vi "ReRouteAroundPolygon.vi"(2 "Desired Point Spacing (in)":dbl, 3 "AvoidancePolygon":T2, 4 "InputPath":T1[](array[typedef])) -> (0 "OutputPath":T1[](array[typedef]), 1 "PathChanged":bool)   [LabVIEW 2017, in "ArgosLib.lvlib"]
uses:
  ArgosLib.lvlib
  TypeDefs/Point2D.ctl
  TypeDefs/Polygon2D.ctl
panel:
  out "Paths":cluster{dbl[], dbl[]}[](graph)
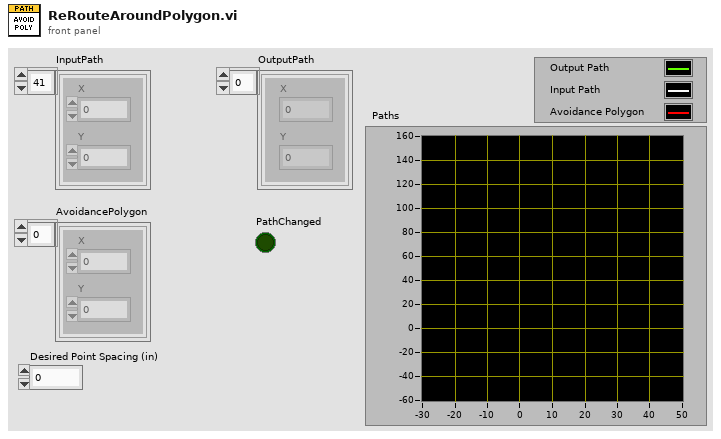
[diagram p1: front panel]
types:
  T1 = typedef "ArgosLib.lvlib/Point2D.ctl" = cluster{"X":dbl, "Y":dbl}
  T2 = typedef "ArgosLib.lvlib/Polygon2D.ctl" = T1[]
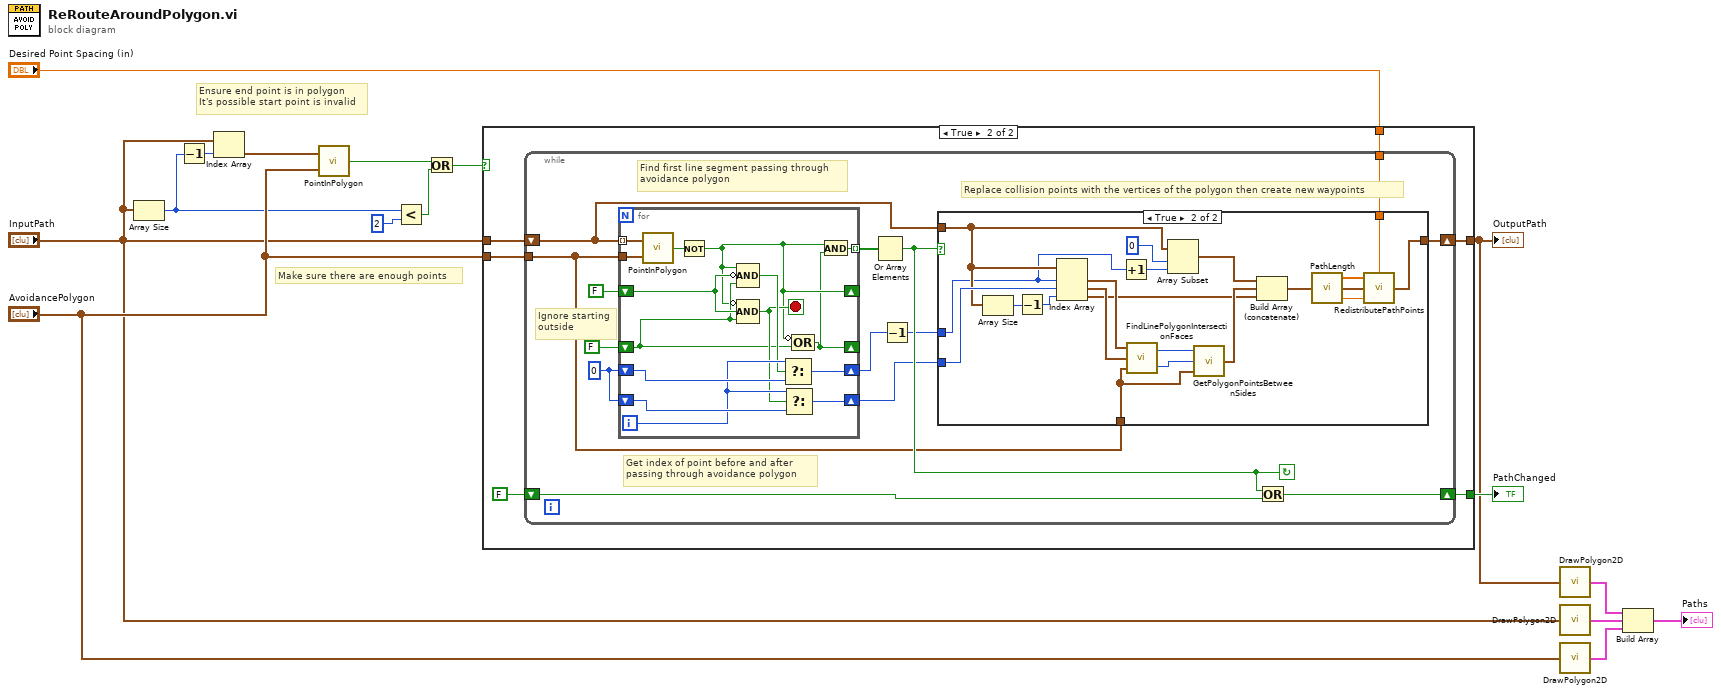
[diagram p0: block diagram]
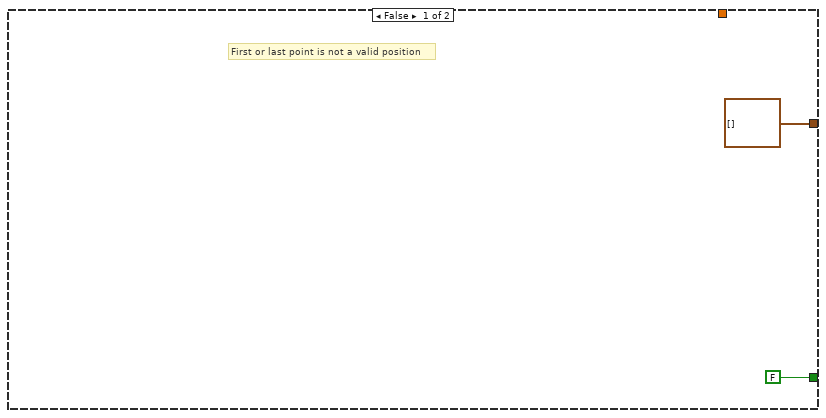
[diagram p2: hidden frame]
diagram:
  # "Ensure end point is in polygon\nIt's possible start point is invalid"
  # "Make sure there are enough points"
  n1 = Array Size(array="InputPath") -> (size(s)=w2:i32)
  n2 = Decrement(x=w2) -> (x-1=w1:i32)
  n3 = Index Array(array="InputPath", index=w1) -> (element=w3:T1)
  n4 = call "PointInPolygon.vi"("Polygon"="AvoidancePolygon", "2DPoint"=w3) -> ("InPolygon"=w4:bool)
  n5 = Less?(x=w2, y=2) -> (x < y?=w13:bool)
  n6 = Or(x=w4, y=w13) -> (x .or. y?=w14:bool)
  n7 = case shown="True" w14 {
    tunnel: [T1[] [] ("InputPath") w24] -> w9
    tunnel: "Desired Point Spacing (in)" -> [_ w22]
    tunnel: [FALSE w21] -> w15
    tunnel: "AvoidancePolygon" -> [_ w20]
    tunnel: "InputPath" -> [_ w19]
    frame False {
      # "First or last point is not a valid position"
    }
    frame True {
      n8 = while {
        tunnel: w20 -> [w28]
        shift-right: [w32] -> w24
        shift-left: w19 -> [w26]
        shift-right: [w36] -> w21
        shift-left: FALSE -> [w35]
        tunnel: w22 -> [w27]
        stop <- w33 continue-if-true
        w34 = 0
        # "Ignore starting\noutside"
        # "Replace collision points with the vertices of the polygon then create new waypoints"
        # "Get index of point before and after\npassing through avoidance polygon"
        # "Find first line segment passing through\navoidance polygon"
        n9 = for {
          tunnel: w26 -> [w65] mode=indexing
          tunnel: w28 -> [w75]
          tunnel: [w62] -> w38 mode=indexing
          shift-right: [w63] -> _
          shift-left: FALSE -> [w74]
          shift-right: [w72] -> w31
          shift-left: w34 -> [w71]
          shift-right: [w70] -> w29
          shift-left: w34 -> [w69]
          shift-right: [w61] -> _
          shift-left: FALSE -> [w64]
          i -> [w68]
          stop <- w66 stop-if-true
          n10 = call "PointInPolygon.vi"("Polygon"=w75, "2DPoint"=w65) -> ("InPolygon"=w73:bool)
          n11 = Not(x=w73) -> (.not. x?=w63:bool)
          n12 = Compound Arithmetic op=AND(w63, invert w74, w64) -> (w67:bool)
          n13 = Compound Arithmetic op=AND(invert w63, w74, w64) -> (w66:bool)
          n14 = Select(t=w68, s=w67, f=w71) -> (s? t:f=w72:i32)
          n15 = Select(t=w68, s=w66, f=w69) -> (s? t:f=w70:i32)
          n16 = Compound Arithmetic op=OR(invert w63, w64) -> (w61:bool)
          n17 = And(x=w63, y=w61) -> (x .and. y?=w62:bool)
        }
        n18 = Or Array Elements(Boolean array=w38) -> (logical OR=w33:bool)
        n19 = Decrement(x=w31) -> (x-1=w30:i32)
        n20 = case shown="True" w33 {
          tunnel: w26 -> [w39 w50]
          tunnel: [w39 w41] -> w32
          tunnel: w30 -> [_ w46]
          tunnel: w29 -> [_ w60]
          tunnel: w28 -> [_ w55]
          tunnel: w27 -> [_ w40]
          frame False {
            # "Path no longer goes through avoidance polygon"
          }
          frame True {
            n21 = Array Size(array=w50) -> (size(s)=w53:i32)
            n22 = Decrement(x=w53) -> (x-1=w52:i32)
            n23 = Index Array(array=w50, index #1=w46, index #2=w60, index #3=w52) -> (element #1=w59:T1, element #2=w58:T1, element #3=w51:T1)
            n24 = Increment(x=w46) -> (x+1=w47:i32)
            n25 = call "FindLinePolygonIntersectionFaces.vi"("Polygon"=w55, "ExitPoint"=w58, "EntryPoint"=w59) -> ("Exit Face"=w56:i32, "Entry Face"=w57:i32)
            n26 = Array Subset(array=w50, index=0, length=w47) -> (w48:T1[])
            n27 = call "GetPolygonPointsBetweenSides.vi"("Polygon"=w55, "LastSideIndex"=w56, "FirstSideIndex"=w57) -> ("PolygonVertices"=w54:T1[])
            n28 = Build Array (concatenate)(w48, w54, w51) -> (w45:T1[])
            n29 = call "PathLength.vi"("PathIn"=w45) -> ("Path Length"=w44:dbl, "PathOut"=w43:T1[], "IndexedPathLength"=w42:dbl[])  [unwired: 2 in]
            n30 = call "RedistributePathPoints.vi"("Desired Point Spacing (in)"=w40, "Path Length (in)"=w44, "PathIn"=w43, "IndexedPathLength"=w42) -> ("PathOut"=w41:T1[])
          }
        }
        n31 = Or(x=w33, y=w35) -> (x .or. y?=w36:bool)
      }
    }
  }
  "OutputPath" <- w9
  "PathChanged" <- w15
  n32 = call "DrawPolygon2D.vi"("Polygon"=w9) -> ("XYPlot"=w8:cluster{dbl[], dbl[]})
  n33 = call "DrawPolygon2D.vi"("Polygon"="InputPath") -> ("XYPlot"=w7:cluster{dbl[], dbl[]})
  n34 = call "DrawPolygon2D.vi"("Polygon"="AvoidancePolygon") -> ("XYPlot"=w6:cluster{dbl[], dbl[]})
  n35 = Build Array(w8, w7, w6) -> (→"Paths":cluster{dbl[], dbl[]}[])
